vi "Calibration_Setup_file.vi"(11 "Path":string) -> ()   [LabVIEW 2019]
uses:
  controls/Data.ctl
  <vilib>/userdefined/High Color/IMAQdx.ctl
  <vilib>/vision/Image Controls.llb/IMAQ Image.ctl
  <vilib>/Utility/config.llb/Write Key (String).vi
  <vilib>/Utility/config.llb/NI_LVConfig.lvlib
panel:
  out "Error Out":errorcluster
  in  "Error In":errorcluster
  in  "input cluster":T1={"L16 Linear Actuator"="", "XE 1000 Pump"="", "Camera1"="", "Camera2"="", "Camera1_IMG"=refnum, "Camera2_IMG"=refnum, "Img_Capt"=FALSE, "Actuator"=FALSE, "Pump"=FALSE, "Cam 1"=FALSE, "Cam 2"=FALSE, "Empty_Refill"=FALSE, "Crop"=FALSE, "Light intensity"=100, "Exposure Time"=1000.0, "Sample Name"="Test Sample", "Operator"="MRJ", "Calibration 1"=path "C:/Users/au540322/Desktop/IHS_Project/images/Debris/Debris_0/Debris_0_2019_06_01-23-32-49-686.PNG", "Calibration 2"=path "C:/Users/au540322/Desktop/IHS_Project/images/Debris/Debris_0/Debris_0_2019_06_01-23-32-49-686.PNG", "Framerate"=1, "Timeout Sample"=50, "Collection date"="MRJ", "Sample size threshold"=1, "Empty start"=1, "Command"="MRJ", "Calibration Image 1"=refnum, "Calibration Image 2"=refnum, "Original Image 1"=refnum, "Original Image 2"=refnum, "Processing Image 1"=refnum, "Processing Image 2"=refnum, "Object Image 1"=refnum, "Object Image 2"=refnum, "Cam 1 - save queue"=refnum, "Cam 2 - save queue"=refnum, "Station"="", "Species Name"="", "Other Notes"="", "Aperture"=enum."Item 0", "Image Process Queue Size"=500, "Image Save Queue Size"=500, "Overload threshold"=500, "Max Framerate"=100, "Blue Plane Image"=refnum, "Subtract Image"=refnum, "Binary Image 1"=refnum, "ROI mask allocation"=refnum, "Rectangle 1"={"Left"=0, "Top"=0, "Right"=0, "Bottom"=0, "Rotation"=0.0}, "Rectangle 2"={"Left"=0, "Top"=0, "Right"=0, "Bottom"=0, "Rotation"=0.0}, "Binary Image 2"=refnum, "Detection Region %"=0.0, "Cam 1 queue"=refnum, "Cam 2 queue"=refnum, "Detect image 1"=refnum, "Detect image 2"=refnum, "Detect 1"=path "C:/Users/au540322/Desktop/IHS_Project/images/Debris/Debris_0/Debris_0_2019_06_01-23-32-49-686.PNG", "Detect 2"=path "C:/Users/au540322/Desktop/IHS_Project/images/Debris/Debris_0/Debris_0_2019_06_01-23-32-49-686.PNG", "Max large object threshold"=0, "Open(T)/Close(F)"=FALSE} {"Rectangle 2"."Rotation" format="%.2f"; "Rectangle 2"."Left" scale=0.0..1024.0; "Rectangle 2"."Right" scale=0.0..1024.0; "Rectangle 1"."Rotation" format="%.2f"; "Rectangle 1"."Left" scale=0.0..1024.0; "Rectangle 1"."Right" scale=0.0..1024.0; "Max Framerate" min=1; "Overload threshold" min=1; "Image Save Queue Size" min=1; "Image Process Queue Size" min=1; "Empty start" min=1; "Sample size threshold" min=1; "Framerate" min=1; "Light intensity" scale=0.0..100.0}
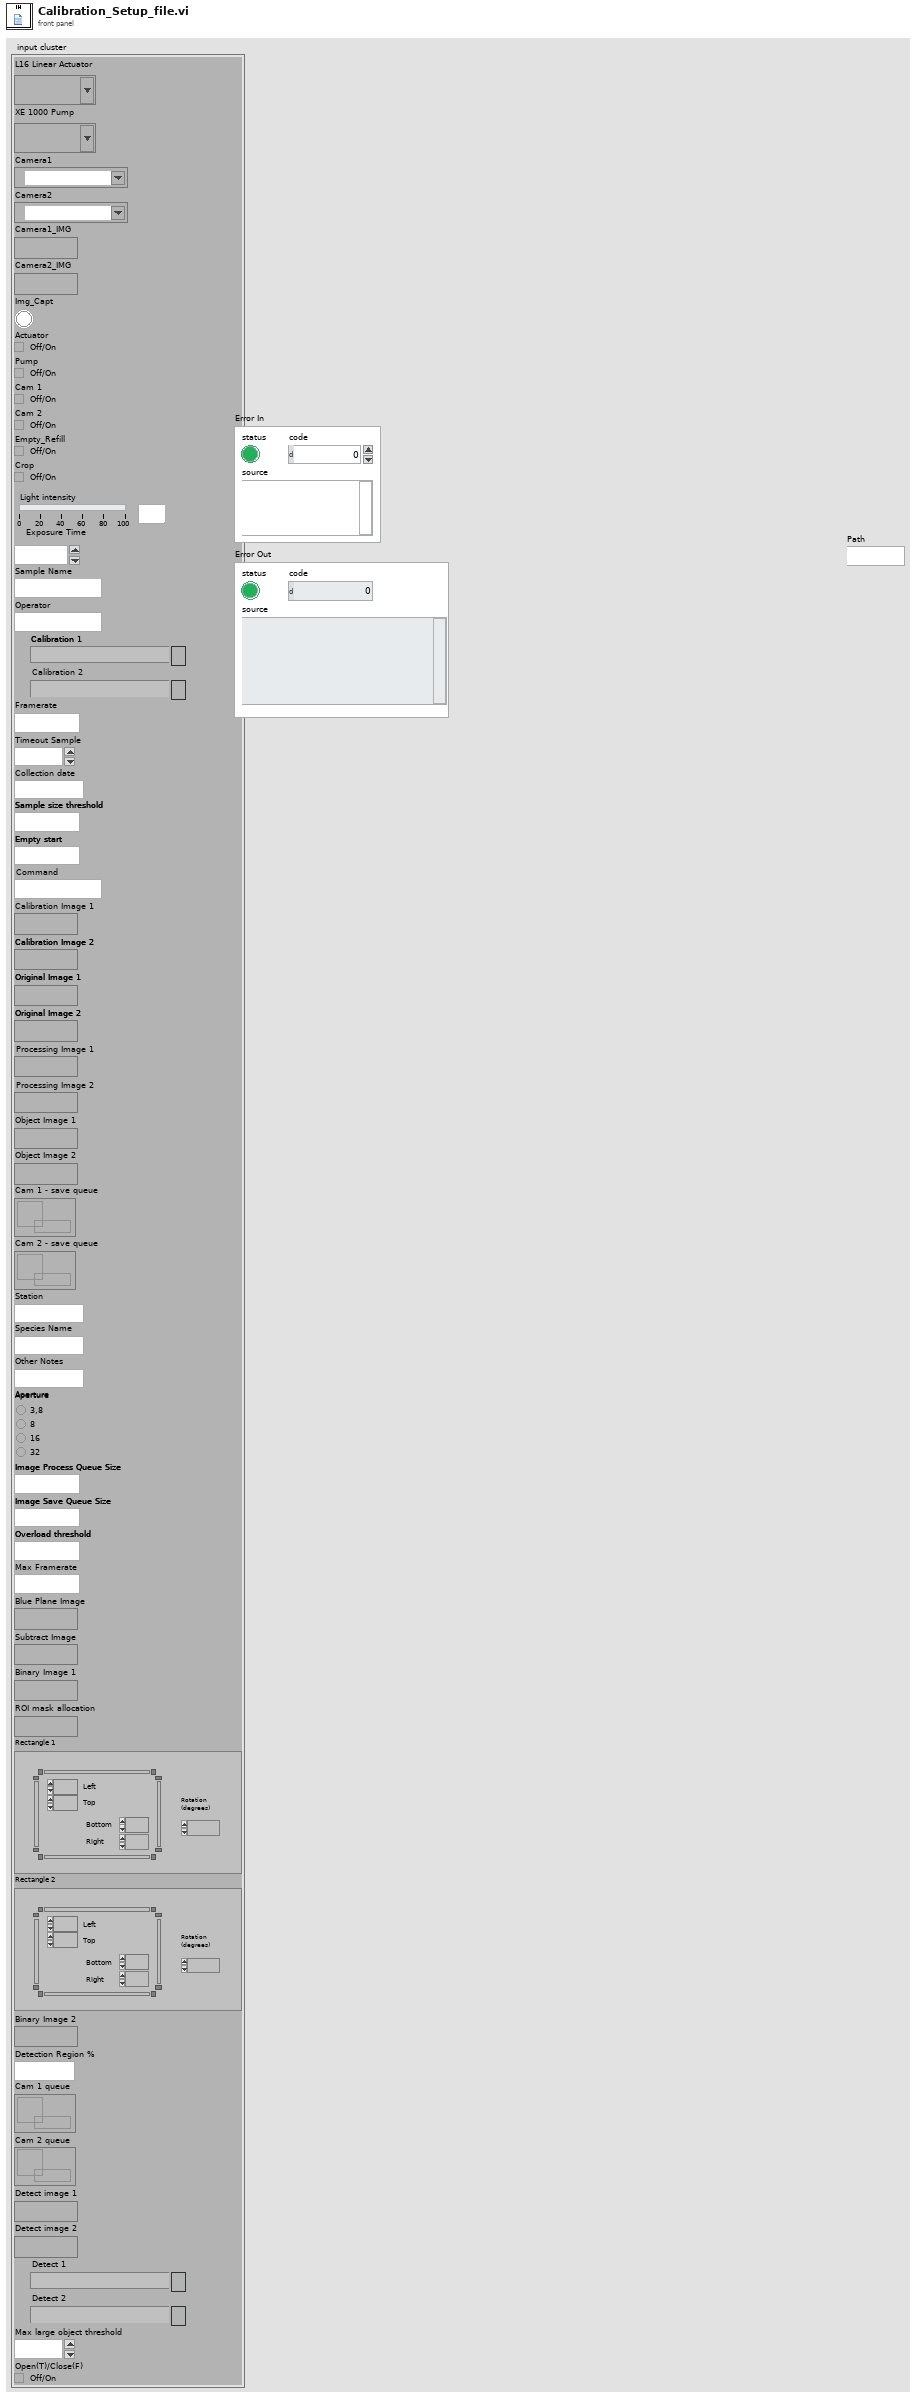
[diagram p1: front panel]
types:
  T1 = typedef "Data.ctl" = cluster{"L16 Linear Actuator":refnum<visa-resource-name>, "XE 1000 Pump":refnum<visa-resource-name>, "Camera1":T2, "Camera2":T2, "Camera1_IMG":T3, "Camera2_IMG":T3, "Img_Capt":bool, "Actuator":bool, "Pump":bool, "Cam 1":bool, "Cam 2":bool, "Empty_Refill":bool, "Crop":bool, "Light intensity":i32, "Exposure Time":dbl, "Sample Name":string, "Operator":string, "Calibration 1":path, "Calibration 2":path, "Framerate":i32, "Timeout Sample":i32, "Collection date":string, "Sample size threshold":i32, "Empty start":u32, "Command":string, "Calibration Image 1":T3, "Calibration Image 2":T3, "Original Image 1":T3, "Original Image 2":T3, "Processing Image 1":T3, "Processing Image 2":T3, "Object Image 1":T3, "Object Image 2":T3, "Cam 1 - save queue":refnum<queue>, "Cam 2 - save queue":refnum<queue>, "Station":string, "Species Name":string, "Other Notes":string, "Aperture":enum32{"Item 0", "Item 1", "Item 2", "Item 3"}, "Image Process Queue Size":i32, "Image Save Queue Size":i32, "Overload threshold":i32, "Max Framerate":i32, "Blue Plane Image":T3, "Subtract Image":T3, "Binary Image 1":T3, "ROI mask allocation":T3, "Rectangle 1":T4, "Rectangle 2":T4, "Binary Image 2":T3, "Detection Region %":dbl, "Cam 1 queue":refnum<queue>, "Cam 2 queue":refnum<queue>, "Detect image 1":T3, "Detect image 2":T3, "Detect 1":path, "Detect 2":path, "Max large object threshold":i32, "Open(T)/Close(F)":bool}
  T2 = typedef "IMAQdx.ctl" = refnum<k21>
  T3 = typedef "IMAQ Image.ctl" = refnum<image>
  T4 = typedef "IMAQ Rectangle" = cluster{"Left":i32, "Top":i32, "Right":i32, "Bottom":i32, "Rotation":dbl}
  T5 = typedef "NI_LVConfig.lvlib/Config Data RefNum.ctl" = refnum<k1>
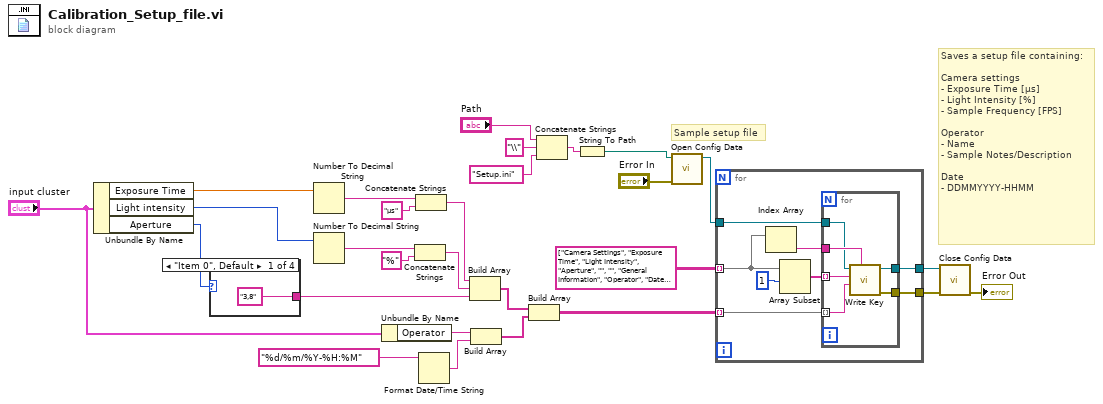
[diagram p0: block diagram]
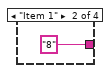
[diagram p2: hidden frame]
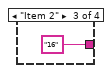
[diagram p3: hidden frame]
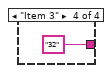
[diagram p4: hidden frame]
diagram:
  # "Saves a setup file containing:\n\nCamera settings\n- Exposure Time [µs]\n- Light Intensity [%]\n- Sample Frequency [FPS]\n\nOperator\n- Name\n- Sample Notes/Description\n\nDate\n- DDMMYYYY-HHMM"
  # "Sample setup file"
  n1 = Unbundle By Name("input cluster") -> ("Exposure Time"=w18:dbl, "Light intensity"=w17:i32, "Aperture"=w6:enum32{"Item 0", "Item 1", "Item 2", "Item 3"})
  n2 = case shown="\"Item 0\", Default" w6 {
    tunnel: ["3,8" "8" "16" "32"] -> w3
    frame "Item 0", Default {
    }
    frame "Item 1" {
    }
    frame "Item 2" {
    }
    frame "Item 3" {
    }
  }
  n3 = Number To Decimal String(number=w18) -> (decimal integer string=w12:string)  [unwired: 1 in]
  n4 = Number To Decimal String(number=w17) -> (decimal integer string=w14:string)  [unwired: 1 in]
  n5 = Unbundle By Name("input cluster") -> ("Operator"=w7:string)
  n6 = Concatenate Strings(w14, "%" ("string")) -> (w13:string)
  n7 = Concatenate Strings(w12, "µs" ("string")) -> (w10:string)
  n8 = Format Date/Time String(time format string (%c)="%d/%m/%Y-%H:%M") -> (date/time string=w2:string)  [unwired: 2 in]
  n9 = Build Array(w10, w13, w3) -> (w28:string[])
  n10 = Build Array(w7, w2) -> (w9:string[])
  n11 = Build Array(w28, w9) -> (w27:string[][])
  n12 = Concatenate Strings("Path", "\\" ("string"), "Setup.ini" ("string")) -> (w21:string)
  n13 = String To Path(string=w21) -> (path=w23:path)
  n14 = call <vilib>:"Open Config Data.vi"("error in (no error)"="Error In", "configuration file path"=w23) -> ("refnum"=w24:T5)  [unwired: 7 in, 2 out]
  n15 = for {
    tunnel: string[][] [["Camera Settings", "Exposure Time", "Light Intensity", "Aperture", "", ""], ["General Information", "Operator", "Date (DD/MM/YYYY)", "", "", ""], ["", "", "", "", "", ""]] ("appended array") -> [w39] mode=indexing
    tunnel: w27 -> [w37] mode=indexing
    tunnel: [w35] -> w26
    tunnel: [w34] -> w25
    tunnel: w24 -> [w33]
    n16 = Index Array(array=w39) -> (element=w38:string)  [unwired: 1 in]
    n17 = Array Subset(array=w39, index=1) -> (w36:string[])  [unwired: 1 in]
    n18 = for {
      tunnel: w38 -> [w46]
      tunnel: w37 -> [w45] mode=indexing
      tunnel: w36 -> [w44] mode=indexing
      tunnel: [w43] -> w35
      tunnel: [w42] -> w34
      tunnel: w33 -> [w41]
      n19 = call-poly <vilib>:"Write Key.vi"("section"=w46, "value"=w45, "key"=w44, "refnum"=w41) -> ("error out"=w42:errorcluster, "refnum out"=w43:T5)  [unwired: 5 in, 1 out]
    }
  }
  n20 = call <vilib>:"Close Config Data.vi"("error in (no error)"=w25, "refnum"=w26) -> ("error out"=→"Error Out":errorcluster)  [unwired: 8 in, 1 out]
